vi "温控状态.vi"(11 "温控状态字":u8) -> (3 "连接的字符串":string)   [LabVIEW 2012]
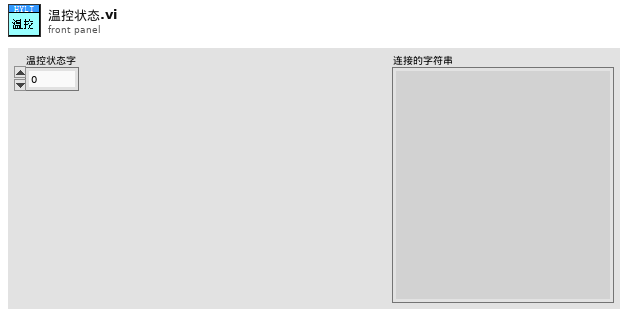
[diagram p1: front panel]
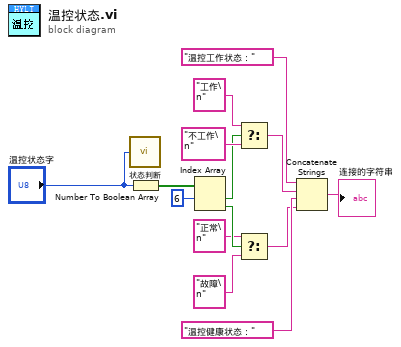
[diagram p0: block diagram]
diagram:
  n1 = call "状态判断.vi"("数值"="温控状态字") -> ()  [unwired: 3 out]
  n2 = Number To Boolean Array(number="温控状态字") -> (Boolean array=w7:bool[])
  n3 = Index Array(array=w7, index #1=6 ("索引")) -> (element #1=w4:bool, element #2=w3:bool)  [unwired: 1 in]
  n4 = Select(t="工作\n" ("主份自检状态及船舱标志"), s=w4, f="不工作\n") -> (s? t:f=w11:string)
  n5 = Select(t="正常\n" ("f"), s=w3, f="故障\n") -> (s? t:f=w9:string)
  n6 = Concatenate Strings("温控工作状态：" ("字符串"), w11, "温控健康状态：" ("字符串"), w9) -> (→"连接的字符串":string)
